vi "gRPC Configuration File Location.vi"() -> (3 "configuration file path":path=path "/home/lvuser/adas_replay_hil/sysconfig/grpc_server.conf")   [LabVIEW 2021, in "gRPC Configuration File.lvlib"]
uses:
  gRPC Configuration File.lvlib
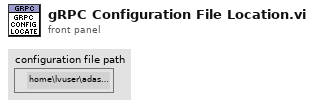
[diagram p1: front panel]
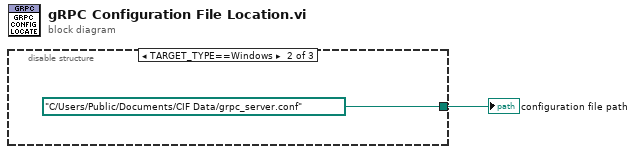
[diagram p0: block diagram]
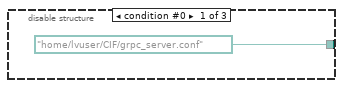
[diagram p2: hidden frame]
diagram:
  n1 = disable-structure shown="TARGET_TYPE==Windows" {
    disable-tunnel: [path "/home/lvuser/CIF/grpc_server.conf" ("configuration file path") path "C:/Users/Public/Documents/CIF Data/grpc_server.conf" ("configuration file path") _] -> w1
    frame condition #0 {
    }
    frame condition #1 (active) {
    }
    frame condition #2 {
    }
  }
  "configuration file path" <- w1
